vi "binary search3VI_Test_as_VI.vi"() -> ()   [LabVIEW 2019]
uses:
  <vilib>/Utility/file.llb/Read Delimited Spreadsheet (DBL).vi
panel:
  in  "Number of\nsamples":dbl=514.0
  in  "X0":sgl=0.5
  out "Waveform Graph 2":dynamicdata(graph)=[{"t0"=timestamp(-0.97 s since 1904-01-01), "dt"=0.06, "Y"=[0.7751937984496124, 2.3255813953488373, 1.550387596899225, 2.3255813953488373, 0.0, 2.3255813953488373, 1.550387596899225, 4.651162790697675, 4.651162790697675, 3.10077519379845, 5.426356589147287, 1.550387596899225, 1.550387596899225, 2.3255813953488373, 1.550387596899225, 3.10077519379845, 5.426356589147287, 0.0, 1.550387596899225, 2.3255813953488373, 0.7751937984496124, 3.10077519379845, 1.550387596899225, 0.7751937984496124, 3.875968992248062, 2.3255813953488373, 2.3255813953488373, 1.550387596899225, 3.875968992248062, 2.3255813953488373, 1.550387596899225, 1.550387596899225, 1.550387596899225, 1.550387596899225, 0.0, 1.550387596899225, 3.10077519379845, 3.10077519379845, 2.3255813953488373, 2.3255813953488373, 0.7751937984496124, 0.7751937984496124, 2.3255813953488373, 1.550387596899225, 0.7751937984496124, 1.550387596899225, 1.550387596899225, 1.550387596899225, 0.0, 0.0], "attributes"=variant("NI_ChannelName"=variant(string " (Histogram)"), "NI_ExpIsRelativeTime"=variant(bool TRUE), "NI_ExpStartTimeStamp"=variant(timestamp timestamp(3682021765.4422193 s since 1904-01-01)), "NI_ExpTimeStamp"=variant(timestamp timestamp(3682021765.4422193 s since 1904-01-01)), "NI_ExpXDimension"=variant(string "BIN"), "NI_OriginalChannelName"=variant(string ""))}]
  out "Histogram":waveform(dbl)(graph)={"t0"=timestamp(0 s since 1904-01-01), "dt"=0.06, "Y"=[0.12919896640826875, 0.3875968992248062, 0.2583979328165375, 0.3875968992248062, 0.0, 0.3875968992248062, 0.2583979328165375, 0.7751937984496124, 0.7751937984496124, 0.516795865633075, 0.9043927648578811, 0.2583979328165375, 0.2583979328165375, 0.3875968992248062, 0.2583979328165375, 0.516795865633075, 0.9043927648578811, 0.0, 0.2583979328165375, 0.3875968992248062, 0.12919896640826875, 0.516795865633075, 0.2583979328165375, 0.12919896640826875, 0.6459948320413437, 0.3875968992248062, 0.3875968992248062, 0.2583979328165375, 0.6459948320413437, 0.3875968992248062, 0.2583979328165375, 0.2583979328165375, 0.2583979328165375, 0.2583979328165375, 0.0, 0.2583979328165375, 0.516795865633075, 0.516795865633075, 0.3875968992248062, 0.3875968992248062, 0.12919896640826875, 0.12919896640826875, 0.3875968992248062, 0.2583979328165375, 0.12919896640826875, 0.2583979328165375, 0.2583979328165375, 0.2583979328165375, 0.0, 0.0]}
  in  "Rg2":sgl=1.0
  out "Waveform Graph":waveform(dbl)(graph)={"t0"=timestamp(0 s since 1904-01-01), "dt"=0.023255813866853714, "Y"=[0.0, 0.0, 0.008396659977734089, 0.016836900264024734, 0.025317199528217316, 0.033834200352430344, 0.04238450154662132, 0.05096510052680969, 0.05957290157675743, 0.06820529699325562, 0.07685939967632294, 0.08553290367126465, 0.09422340244054794, 0.1029290035367012, 0.11164700239896774, 0.12037599831819534, 0.12911400198936462, 0.13785900175571442, 0.14661100506782532, 0.15536700189113617, 0.16412599384784698, 0.17288799583911896, 0.18165099620819092, 0.19041499495506287, 0.19917799532413483, 0.2079409956932068, 0.21670199930667877, 0.22546100616455078, 0.23421800136566162, 0.2429720014333725, 0.2517240047454834, 0.26047199964523315, 0.26921799778938293, 0.27796098589897156, 0.2867009937763214, 0.2954379916191101, 0.30417200922966003, 0.3129050135612488, 0.32163500785827637, 0.330363005399704, 0.3390899896621704, 0.34781599044799805, 0.3565410077571869, 0.36526501178741455, 0.373989999294281, 0.38271400332450867, 0.3914400041103363, 0.40016600489616394, 0.40889400243759155, 0.41762399673461914, 0.4263559877872467, 0.4350909888744354, 0.4438279867172241, 0.4525670111179352, 0.4613099992275238, 0.47005701065063477, 0.4788059890270233, 0.4875589907169342, 0.49631598591804504, 0.5050749778747559, 0.5138369798660278, 0.5226029753684998, 0.531370997428894, 0.5401399731636047, 0.548911988735199, 0.5576840043067932, 0.5664560198783875, 0.5752279758453369, 0.5839980244636536, 0.5927659869194031, 0.6015300154685974, 0.6102880239486694, 0.6190400123596191, 0.627784013748169, 0.6365180015563965, 0.6452410221099854, 0.6539490222930908, 0.6626420021057129, 0.6713169813156128, 0.6799709796905518, 0.6886019706726074, 0.6972060203552246, 0.7057819962501526, 0.714326024055481, 0.7228350043296814, 0.7313050031661987, 0.7397329807281494, 0.7481160163879395, 0.7564489841461182, 0.7647280097007751, 0.7729489803314209, 0.7811089754104614, 0.7892029881477356, 0.7972260117530823, 0.8051739931106567, 0.8130419850349426, 0.82082599401474, 0.8285199999809265, 0.8361210227012634, 0.8436229825019836, 0.8510220050811768, 0.8583109974861145, 0.8654879927635193, 0.8725469708442688, 0.8794829845428467, 0.8862910270690918, 0.8929679989814758, 0.899507999420166, 0.9059079885482788, 0.9121630191802979, 0.9182699918746948, 0.9242249727249146, 0.9300230145454407, 0.9356629848480225, 0.9411410093307495, 0.9464550018310547, 0.9516019821166992, 0.9565799832344055, 0.9613879919052124, 0.9660239815711975, 0.9704869985580444, 0.9747779965400696, 0.9788950085639954, 0.9828389883041382, 0.9866099953651428, 0.990211009979248, 0.9936410188674927, 0.9969030022621155, 1.0]}
  in  "RG factor":dbl=1.0
  in  "right domain":sgl=18.0
  out "size(s) 2":i32=130
  out "Array":sgl[](array[numeric])=[0.0, 0.0, 0.0, 0.00839666, 0.0168369, 0.0253172, 0.0338342, 0.0423845, 0.0509651, 0.0595729, 0.0682053, 0.0768594, 0.0855329, 0.0942234, 0.102929, 0.111647, 0.120376, 0.129114, 0.137859, 0.146611, 0.155367, 0.164126, 0.172888, 0.181651, 0.190415, 0.199178, 0.207941, 0.216702, 0.225461, 0.234218, 0.242972, 0.251724, 0.260472, 0.269218, 0.277961, 0.286701, 0.295438, 0.304172, 0.312905, 0.321635, 0.330363, 0.33909, 0.347816, 0.356541, 0.365265, 0.37399, 0.382714, 0.39144, 0.400166, 0.408894, 0.417624, 0.426356, 0.435091, 0.443828, 0.452567, 0.46131, 0.470057, 0.478806, 0.487559, 0.496316, 0.505075, 0.513837, 0.522603, 0.531371, 0.54014, 0.548912, 0.557684, 0.566456, 0.575228, 0.583998, 0.592766, 0.60153, 0.610288, 0.61904, 0.627784, 0.636518, 0.645241, 0.653949, 0.662642, 0.671317, 0.679971, 0.688602, 0.697206, 0.705782, 0.714326, 0.722835, 0.731305, 0.739733, 0.748116, 0.756449, 0.764728, 0.772949, 0.781109, 0.789203, 0.797226, 0.805174, 0.813042, 0.820826, 0.82852, 0.836121, 0.843623, 0.851022, 0.858311, 0.865488, 0.872547, 0.879483, 0.886291, 0.892968, 0.899508, 0.905908, 0.912163, 0.91827, 0.924225, 0.930023, 0.935663, 0.941141, 0.946455, 0.951602, 0.95658, 0.961388, 0.966024, 0.970487, 0.974778, 0.978895, 0.982839, 0.98661, 0.990211, 0.993641, 0.996903, 1.0] format="%.6f"
  out "Init Data Out":sgl[](array[numeric])=[0.0, 0.0, 0.00839666, 0.0168369, 0.0253172, 0.0338342, 0.0423845, 0.0509651, 0.0595729, 0.0682053, 0.0768594, 0.0855329, 0.0942234, 0.102929, 0.111647, 0.120376, 0.129114, 0.137859, 0.146611, 0.155367, 0.164126, 0.172888, 0.181651, 0.190415, 0.199178, 0.207941, 0.216702, 0.225461, 0.234218, 0.242972, 0.251724, 0.260472, 0.269218, 0.277961, 0.286701, 0.295438, 0.304172, 0.312905, 0.321635, 0.330363, 0.33909, 0.347816, 0.356541, 0.365265, 0.37399, 0.382714, 0.39144, 0.400166, 0.408894, 0.417624, 0.426356, 0.435091, 0.443828, 0.452567, 0.46131, 0.470057, 0.478806, 0.487559, 0.496316, 0.505075, 0.513837, 0.522603, 0.531371, 0.54014, 0.548912, 0.557684, 0.566456, 0.575228, 0.583998, 0.592766, 0.60153, 0.610288, 0.61904, 0.627784, 0.636518, 0.645241, 0.653949, 0.662642, 0.671317, 0.679971, 0.688602, 0.697206, 0.705782, 0.714326, 0.722835, 0.731305, 0.739733, 0.748116, 0.756449, 0.764728, 0.772949, 0.781109, 0.789203, 0.797226, 0.805174, 0.813042, 0.820826, 0.82852, 0.836121, 0.843623, 0.851022, 0.858311, 0.865488, 0.872547, 0.879483, 0.886291, 0.892968, 0.899508, 0.905908, 0.912163, 0.91827, 0.924225, 0.930023, 0.935663, 0.941141, 0.946455, 0.951602, 0.95658, 0.961388, 0.966024, 0.970487, 0.974778, 0.978895, 0.982839, 0.98661, 0.990211, 0.993641, 0.996903, 1.0]
  out "Time_delay":dbl=0.001970199984498322
  out "size(s)":i32=129
  out "Waveform Chart":sgl[](graph)=[-0.5007627, -0.26172853, -0.9675348, -0.79714173, -0.8499071, -0.4081716, -0.67888236, 0.8678531, 1.340557, -0.12069799, -0.053550687, -0.7712974, -0.9118137, 0.46712488, 0.60156405, 1.2902113, 1.8243805, 0.5856648, -0.4015777, 1.5688123, 0.91011286, -0.37849522, -0.66814816, -0.06282105, -0.042828422, 0.016113404, 1.2304785, 1.2057705, 0.74746245, -0.34551492, -0.1558953, 0.9642982, 0.0092038885, 0.00058439746, -0.50516504, -0.79901195, 0.72839165, 1.5293171, -0.6899687, 1.7245603, 1.6015321, 0.09580641, -0.533587, 0.3736991, 1.2313154, -0.86675215, -0.3698279, 0.92464036, -0.24675827, 1.0315081, -0.4358851, 1.7305485, 1.00724, -0.49945712, -0.62267965, 0.5650846, -0.3407286, 0.14589624, 1.7849993, 0.8405116, 1.1729848, 0.77362686, 1.4353051, -0.5409261, -0.3202128, -0.5514956, -0.09313411, 0.69906884, 1.4973538, 0.44492182, -0.0072780503, 0.72927696, 1.2549423, -0.90609664, 0.36230835, -0.3731676, -0.4746058, -0.35410124, 0.82364136, 1.1128618, 1.8425759, 0.7174704, -0.5618813, -0.49711367, 0.44848984, -0.57690513, 0.19557971, 0.7315942, -0.035114788, -0.21315603, 0.4731006, 1.2657732, -0.34774807, -0.21388197, -0.924264, 1.6178749, 0.64356995, -0.29602507, 1.6704447, 1.171573, 0.5502283, 0.7929559, 0.29514176, 0.28289402, 0.2926584, -0.44214937, 1.1886274, 0.13503134, 1.5481986, -0.19797295, 0.31180936, -0.51264226, 1.3716698, -0.6255967, 1.3509319, 1.2978759, 0.50538135, -0.5749768, 0.48093557, 0.18186033, 1.7823807, 0.54670197, -0.00055433536, 1.3052928, 0.41797948, 1.1314512, -0.0086068, 0.6392585, 0.2218753]
  in  "Cold":path=path "C:/Users/Diffusivity/OneDrive - sfu.ca/Mpemba/InvMpemba/cum for InvMP/Tb=1/T1.0.txt"
  # "Only change this to not be equal to size(s) if you want to test that the \nhistograms are okay. size(s) 2 should be equal to size(s) if modifying FPGA"
  # "This should be 18 for \nregular Mpemba experiments"
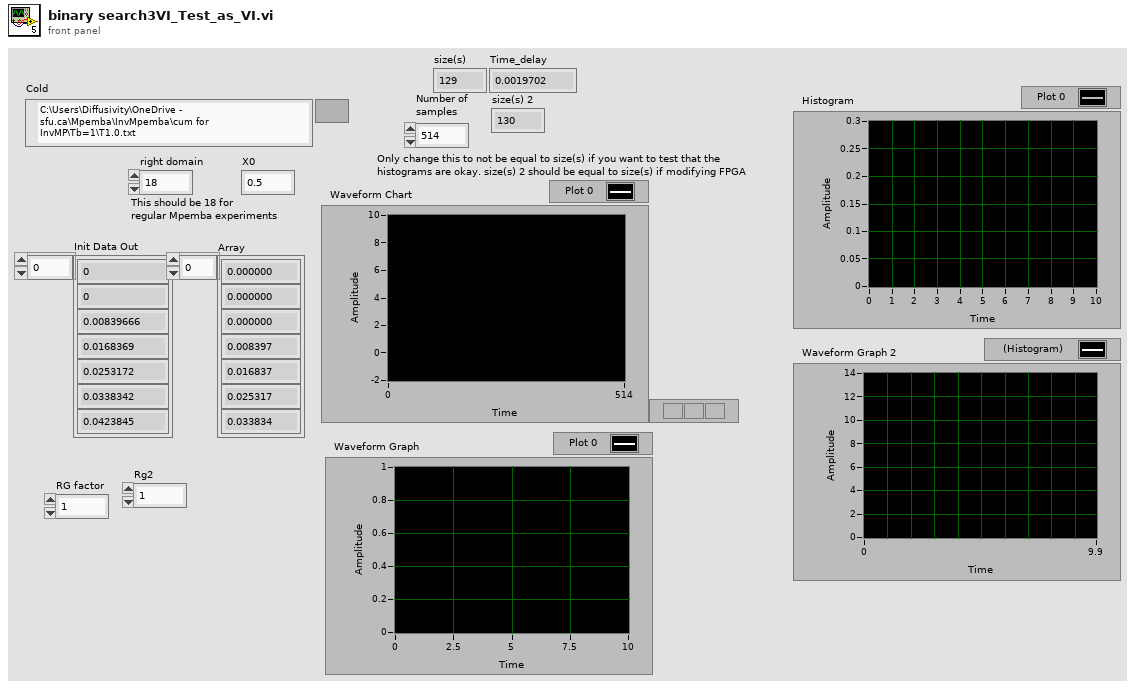
[diagram p1: front panel]
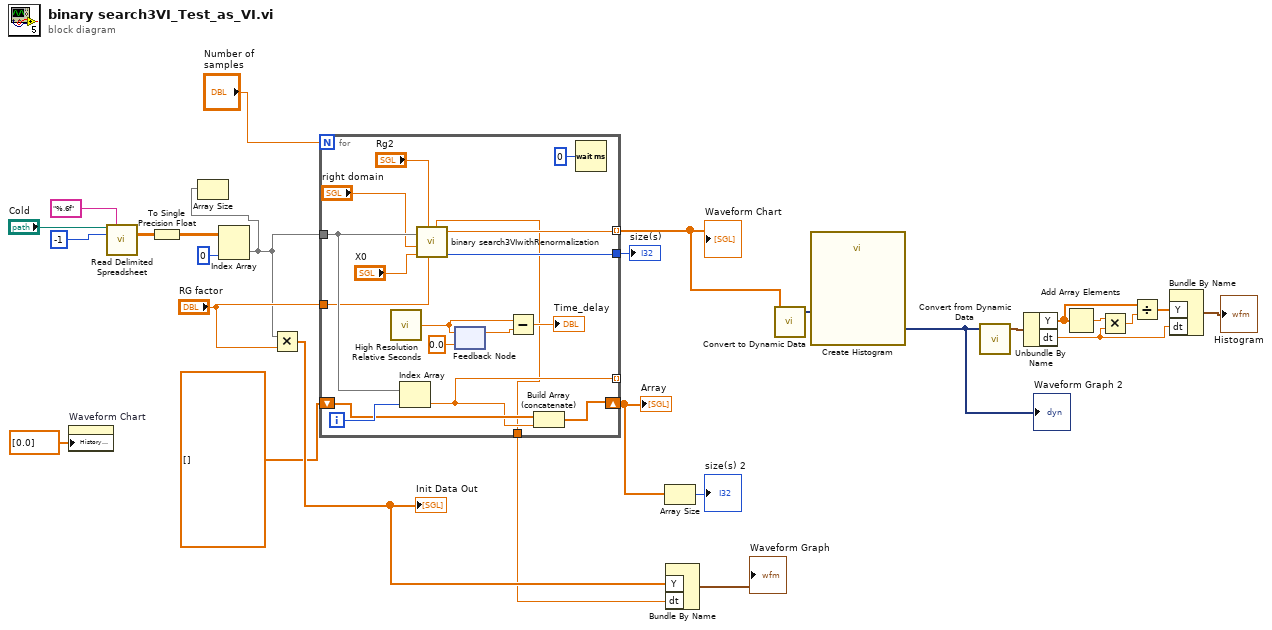
[diagram p0: block diagram]
diagram:
  n1 = property on="Waveform Chart" class="WFChart (strict)"("History Data"=dbl[] [0.0]) -> ()  [unwired: 2 in, 2 out]
  n2 = call-poly <vilib>:"Read Delimited Spreadsheet.vi"("file path (dialog if empty)"="Cold", "format (%.3f)"="%.6f", "number of rows (all:-1)"=-1) -> ("all rows"=w19:dbl[][])  [unwired: 7 in, 5 out]
  n3 = To Single Precision Float(number=w19) -> (single precision float=w22:sgl[][])
  n4 = Index Array(array=w22, index (col)=0 ("disabled index (col)")) -> (element=w4:sgl[])  [unwired: 1 in]
  n5 = Array Size(array=w4) -> ()  [unwired: 1 out]
  n6 = Multiply(x=w4, y="RG factor") -> (x*y=w15:dbl[])
  "Init Data Out" <- w15
  n7 = for {
    N: "Number of\nsamples" -> [_]
    tunnel: w4 -> [w37]
    tunnel: [w43] -> w12 mode=indexing
    tunnel: [w42] -> w24
    shift-right: [w34] -> w18
    shift-left: sgl[] [] -> [w35]
    tunnel: [w33] -> _ mode=indexing
    tunnel: "RG factor" -> [w31]
    tunnel: [w30] -> w14
    i -> [w36]
    n8 = call <vilib>:"High Resolution Relative Seconds.vi"() -> ("relative seconds"=w40:dbl)
    n9 = Index Array(array=w37, index=w36) -> (element=w33:sgl)
    n10 = call "binary search3VIwithRenormalization.vi"("Renormalization Factor"=w31, "Rg2"="Rg2", "X0"="X0", "right domain"="right domain", "array"=w37) -> ("size(s)"=w42:i32, "Xpot"=w43:sgl, "dx"=w30:sgl)  [unwired: 2 in, 2 out]
    n11 = feedback-in #1(w40) -> ()
    n12 = feedback #1(0.0 ("relative seconds")) -> (w39:dbl)
    n13 = Subtract(x=w40, y=w39) -> (x-y=→"Time_delay":dbl)
    n14 = Build Array (concatenate)(w35, w33) -> (w34:sgl[])
    n15 = Wait (ms)(milliseconds to wait=u32 0) -> ()  [unwired: 1 out]
  }
  "size(s)" <- w24
  "Waveform Chart" <- w12
  "Array" <- w18
  n16 = Array Size(array=w18) -> (size(s)=→"size(s) 2":i32)
  n17 = Bundle By Name("Y"=w15, "dt"=w14) -> (→"Waveform Graph":waveform(dbl))  [unwired: 1 in]
  n18 = call "Convert to Dynamic Data"("Array"=w12) -> ("Dynamic Data Type"=w16:dynamicdata)  [unwired: 3 in]
  n19 = call "Create Histogram"("Signal"=w16) -> ("Histogram"=w3:dynamicdata)  [unwired: 9 in, 1 out]
  "Waveform Graph 2" <- w3
  n20 = call "Convert from Dynamic Data"("Dynamic Data Type"=w3) -> ("Waveform"=w11:waveform(dbl))  [unwired: 3 in]
  n21 = Unbundle By Name(w11) -> ("Y"=w9:dbl[], "dt"=w6:dbl)
  n22 = Add Array Elements(numeric array=w9) -> (sum=w10:dbl)
  n23 = Multiply(x=w10, y=w6) -> (x*y=w8:dbl)
  n24 = Divide(x=w9, y=w8) -> (x/y=w7:dbl[])
  n25 = Bundle By Name("Y"=w7, "dt"=w6) -> (→"Histogram":waveform(dbl))  [unwired: 1 in]
